vi "Check File Path 2012 NIVerified.vi"(8 "error in":errorcluster, 11 "Path to Check":path) -> (0 "error out":errorcluster, 1 "Path Modified?":bool, 2 "Original Path":path, 3 "Valid Path":path)   [LabVIEW 2022 SP3]
panel:
  # "Inputs"
  # "Outputs"
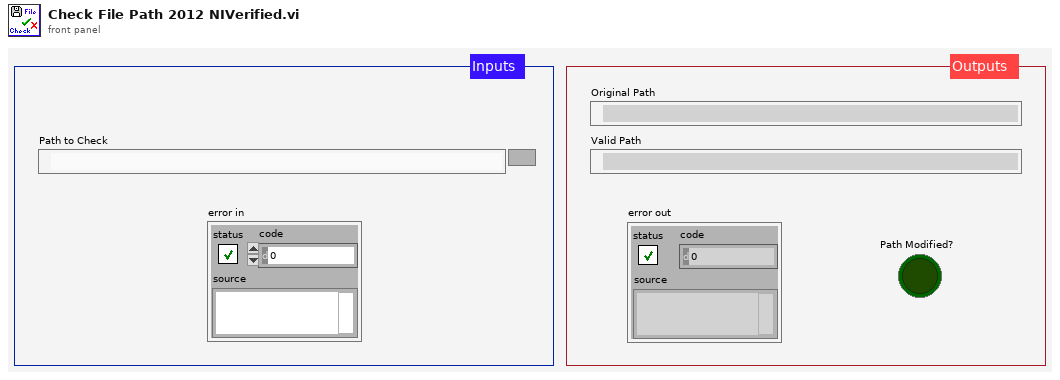
[diagram p1: front panel]
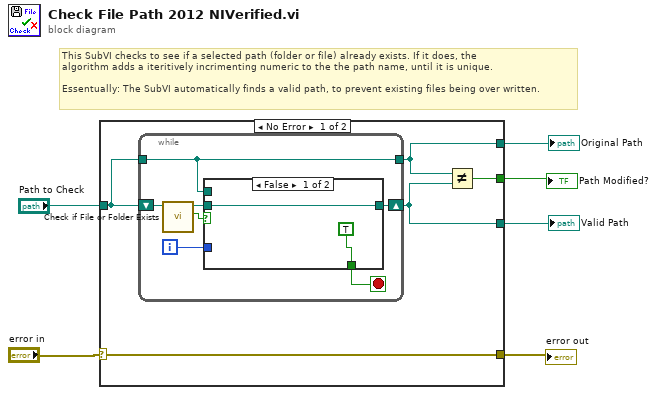
[diagram p0: block diagram]
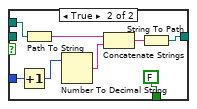
[diagram p2: hidden frame]
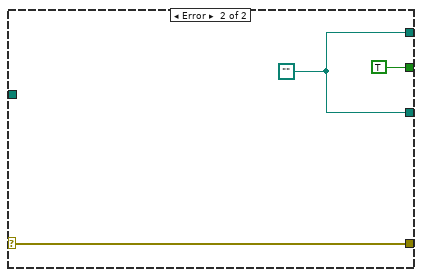
[diagram p3: hidden frame]
diagram:
  # "This SubVI checks to see if a selected path (folder or file) already exists. If it does, the \nalgorithm adds a iteritively incrimenting numeric to the the path name, until it is unique.\n\nEssentually: The SubVI automatically finds a valid path, to prevent existing files being over written."
  n1 = case shown="No Error" "error in" {
    selector: "error in" -> [w8 w30]
    tunnel: "Path to Check" -> [w7 _]
    tunnel: [w11 w29] -> w5
    tunnel: [w10 w29] -> w4
    tunnel: [w9 TRUE] -> w3
    tunnel: [w8 w30] -> w1
    frame No Error {
      n2 = while {
        shift-right: [w16] -> w10
        shift-left: w7 -> [w15]
        tunnel: [w13] -> w11
        tunnel: w7 -> [w13]
        i -> [w14]
        stop <- w17 stop-if-true
        n3 = call <vilib>:"Check if File or Folder Exists.vi"("path"=w15) -> ("file or folder exists?"=w18:bool, "dup path"=w12:path)  [unwired: 8 in, 1 out]
        n4 = case shown="False" w18 {
          tunnel: w13 -> [_ w28]
          tunnel: [TRUE FALSE] -> w17
          tunnel: w14 -> [_ w27]
          tunnel: [w19 w23] -> w16
          tunnel: w12 -> [w19 _]
          frame False {
          }
          frame True {
            n5 = Increment(x=w27) -> (x+1=w21:i32)
            n6 = Path To String(path=w28) -> (string=w26:string)
            n7 = Number To Decimal String(number=w21) -> (decimal integer string=w25:string)  [unwired: 1 in]
            n8 = Concatenate Strings(w26, w25) -> (w24:string)
            n9 = String To Path(string=w24) -> (path=w23:path)
          }
        }
      }
      n10 = Not Equal?(x=w11, y=w10) -> (x != y?=w9:bool)
    }
    frame Error {
      w29 = path ""
    }
  }
  "Valid Path" <- w4
  "Path Modified?" <- w3
  "Original Path" <- w5
  "error out" <- w1
